vi "JOYSTICK MANUAL SUBVI.vi"   [LabVIEW 2013]
uses:
  <vilib>/Rock Robotics/WPI/Joystick/WPI_JoystickGetSetRefNum.vi
types:
  T1 = typedef "WPI_JoystickDevRef.ctl" = cluster{"Device":T2}
  T2 = typedef "WPI_JoystickDeviceEnum.ctl" = enum16{"USB 1", "USB 2", "USB 3", "USB 4", "Kinect 1", "Kinect 2"}
  T3 = cluster{"axis 1 (x)":dbl, "axis 2 (y)":dbl, "axis 3 (throttle)":dbl, "axis 4":dbl, "axis 5":dbl, "axis 6":dbl}
  T4 = typedef "WPI_JoystickButtonState.ctl" = cluster{"Button 1":bool, "Button 2":bool, "Button 3":bool, "Button 4":bool, "Button 5":bool, "Button 6":bool, "Button 7":bool, "Button 8":bool, "Button 9":bool, "Button 10":bool, "Button 11":bool, "Button 12":bool}
  T5 = typedef "WPI_MotorControlDeviceRef.ctl" = cluster{"DeviceStatus":errorcluster, "Type":enum16{"PWM", "CAN"}, "PWM":cluster{"Digital Module":T6, "PWM Channel":T7, "DeadBand":T8}, "CAN":cluster{"Device Number":u8, "Control Mode":T9, "Semaphore":T10, "Max Vout":dbl}, "Invert":bool, "TransformRef":T11, "InvTransformRef":T11}
  T6 = typedef "FPGA_TypedefDigitalModule.ctl" = enum16{"Digital Module 1", "Digital Module 2"}
  T7 = typedef "FPGA_DIOPWMChannel.ctl" = enum8{"PWM 1", "PWM 2", "PWM 3", "PWM 4", "PWM 5", "PWM 6", "PWM 7", "PWM 8", "PWM 9", "PWM 10", "Invalid"}
  T8 = typedef "WPI_PWMDeadband.ctl" = cluster{"Name":string, "maxPositivePwm":i32, "minPositivePwm":i32, "centerPwm":i32, "maxNegativePwm":i32, "minNegativePwm":i32, "angularRange":u16}
  T9 = typedef "WPI_CANJaguar_ControlMode.ctl" = enum8{"Percent VBus", "Current", "Speed", "Position", "Voltage"}
  T10 = typedef "Semaphore RefNum" = refnum<k1>
  T11 = typedef "WPI_PWMTransform_ConPane.ctl" = refnum<vi>
  T12 = typedef "WPI_DigitalInputDevRef.ctl" = cluster{"DevStatus":errorcluster, "DIO Channel":T13, "Digital Module":T6}
  T13 = typedef "FPGA_DIOChannel.ctl" = enum8{"DIO 1", "DIO 2", "DIO 3", "DIO 4", "DIO 5", "DIO 6", "DIO 7", "DIO 8", "DIO 9", "DIO 10", "DIO 11", "DIO 12", "DIO 13", "DIO 14", "Invalid"}
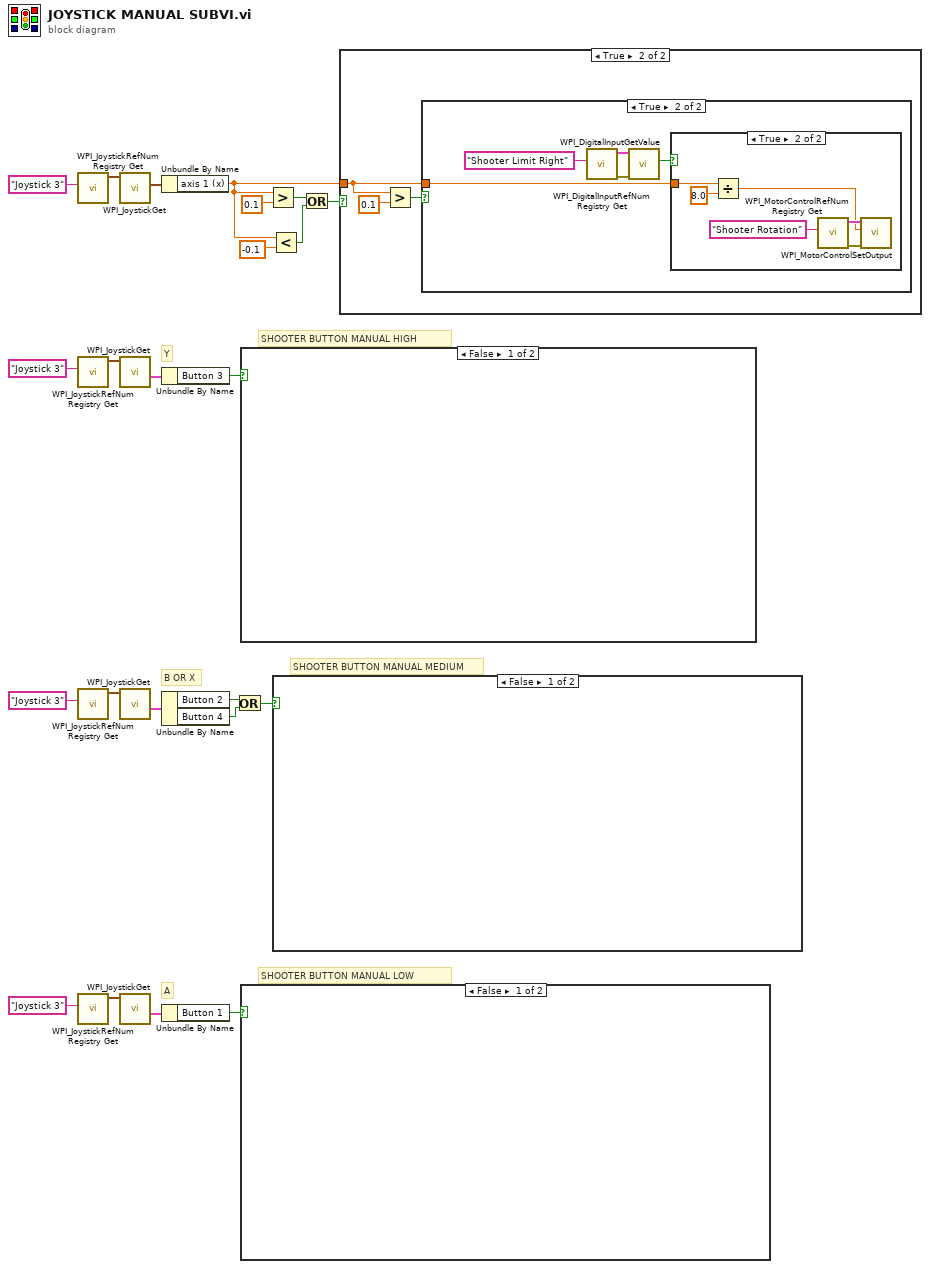
[diagram p0: block diagram]
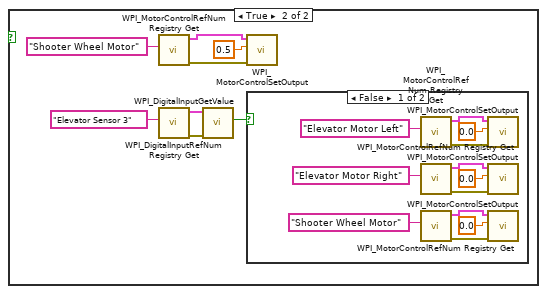
[diagram p2: hidden frame]
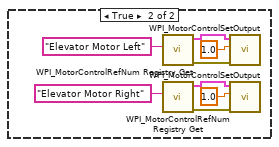
[diagram p3: hidden frame]
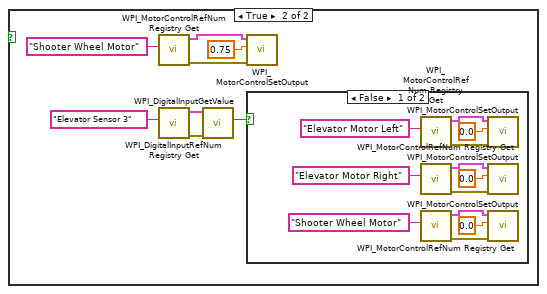
[diagram p4: hidden frame]
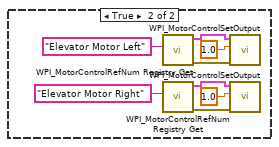
[diagram p5: hidden frame]
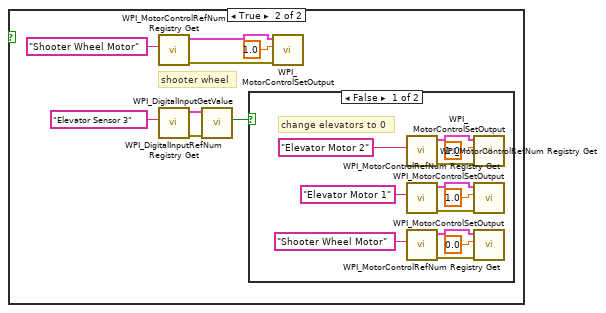
[diagram p6: hidden frame]
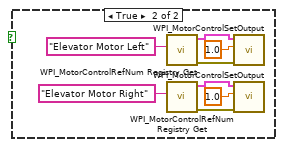
[diagram p7: hidden frame]
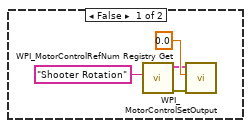
[diagram p8: hidden frame]
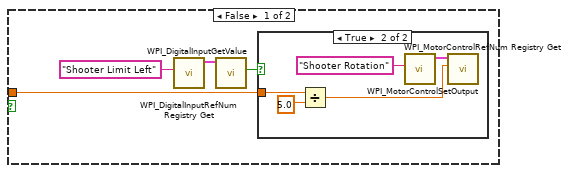
[diagram p9: hidden frame]
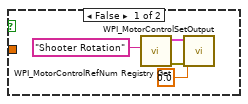
[diagram p10: hidden frame]
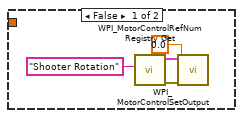
[diagram p11: hidden frame]
diagram:
  # "A"
  # "SHOOTER BUTTON MANUAL LOW"
  # "B OR X"
  # "SHOOTER BUTTON MANUAL MEDIUM"
  # "Y"
  # "SHOOTER BUTTON MANUAL HIGH"
  n1 = call <vilib>:"WPI_JoystickRefNum Registry Get.vi"("refnum name"="Joystick 3") -> ("JoystickDevRef"=w15:T1)  [unwired: 9 in, 1 out]
  n2 = call <vilib>:"WPI_JoystickRefNum Registry Get.vi"("refnum name"="Joystick 3") -> ("JoystickDevRef"=w14:T1)  [unwired: 9 in, 1 out]
  n3 = call <vilib>:"WPI_JoystickRefNum Registry Get.vi"("refnum name"="Joystick 3") -> ("JoystickDevRef"=w10:T1)  [unwired: 9 in, 1 out]
  n4 = call <vilib>:"WPI_JoystickRefNum Registry Get.vi"("refnum name"="Joystick 3") -> ("JoystickDevRef"=w4:T1)  [unwired: 9 in, 1 out]
  n5 = call <vilib>:"WPI_JoystickGet.vi"("JoystickDevRef"=w15) -> ("Axes"=w17:T3)  [unwired: 4 in, 2 out]
  n6 = call <vilib>:"WPI_JoystickGet.vi"("JoystickDevRef"=w14) -> ("Buttons"=w13:T4)  [unwired: 4 in, 2 out]
  n7 = call <vilib>:"WPI_JoystickGet.vi"("JoystickDevRef"=w10) -> ("Buttons"=w8:T4)  [unwired: 4 in, 2 out]
  n8 = call <vilib>:"WPI_JoystickGet.vi"("JoystickDevRef"=w4) -> ("Buttons"=w2:T4)  [unwired: 4 in, 2 out]
  n9 = Unbundle By Name(w17) -> ("axis 1 (x)"=w21:dbl)
  n10 = Unbundle By Name(w13) -> ("Button 3"=w12:bool)
  n11 = Unbundle By Name(w8) -> ("Button 2"=w7:bool, "Button 4"=w6:bool)
  n12 = Unbundle By Name(w2) -> ("Button 1"=w1:bool)
  n13 = Or(x=w7, y=w6) -> (x .or. y?=w5:bool)
  n14 = case shown="False" w12 {
    frame False {
    }
    frame True {
      # "shooter wheel"
      n15 = call <vilib>:"WPI_MotorControlRefNum Registry Get.vi"("refnum name"="Shooter Wheel Motor") -> ("error out"=w27:errorcluster, "MotorControlDevRef"=w26:T5)  [unwired: 9 in]
      n16 = call <vilib>:"WPI_DigitalInputRefNum Registry Get.vi"("refnum name"="Elevator Sensor 3") -> ("error out"=w30:errorcluster, "DigitalInputDevRef"=w29:T12)  [unwired: 9 in]
      n17 = call <vilib>:"WPI_DigitalInputGetValue.vi"("error in (no error)"=w30, "DigitalInputDevRef"=w29) -> ("Value"=w28:bool)  [unwired: 7 in, 2 out]
      n18 = case shown="False" w28 {
        frame False {
          # "change elevators to 0"
          n19 = call <vilib>:"WPI_MotorControlRefNum Registry Get.vi"("refnum name"="Elevator Motor 2") -> ("error out"=w43:errorcluster, "MotorControlDevRef"=w42:T5)  [unwired: 9 in]
          n20 = call <vilib>:"WPI_MotorControlRefNum Registry Get.vi"("refnum name"="Elevator Motor 1") -> ("error out"=w39:errorcluster, "MotorControlDevRef"=w38:T5)  [unwired: 9 in]
          n21 = call <vilib>:"WPI_MotorControlRefNum Registry Get.vi"("refnum name"="Shooter Wheel Motor") -> ("error out"=w35:errorcluster, "MotorControlDevRef"=w34:T5)  [unwired: 9 in]
          n22 = call <vilib>:"WPI_MotorControlSetOutput.vi"("error in (no error)"=w43, "Output"=1.0, "MotorControlDevRef"=w42) -> ()  [unwired: 6 in, 3 out]
          n23 = call <vilib>:"WPI_MotorControlSetOutput.vi"("error in (no error)"=w39, "Output"=1.0, "MotorControlDevRef"=w38) -> ()  [unwired: 6 in, 3 out]
          n24 = call <vilib>:"WPI_MotorControlSetOutput.vi"("error in (no error)"=w35, "Output"=0.0, "MotorControlDevRef"=w34) -> ()  [unwired: 6 in, 3 out]
        }
        frame True {
          n25 = call <vilib>:"WPI_MotorControlRefNum Registry Get.vi"("refnum name"="Elevator Motor Left") -> ("error out"=w51:errorcluster, "MotorControlDevRef"=w50:T5)  [unwired: 9 in]
          n26 = call <vilib>:"WPI_MotorControlRefNum Registry Get.vi"("refnum name"="Elevator Motor Right") -> ("error out"=w47:errorcluster, "MotorControlDevRef"=w46:T5)  [unwired: 9 in]
          n27 = call <vilib>:"WPI_MotorControlSetOutput.vi"("error in (no error)"=w51, "Output"=1.0, "MotorControlDevRef"=w50) -> ()  [unwired: 6 in, 3 out]
          n28 = call <vilib>:"WPI_MotorControlSetOutput.vi"("error in (no error)"=w47, "Output"=1.0, "MotorControlDevRef"=w46) -> ()  [unwired: 6 in, 3 out]
        }
      }
      n29 = call <vilib>:"WPI_MotorControlSetOutput.vi"("error in (no error)"=w27, "Output"=1.0, "MotorControlDevRef"=w26) -> ()  [unwired: 6 in, 3 out]
    }
  }
  n30 = case shown="False" w1 {
    frame False {
    }
    frame True {
      n31 = call <vilib>:"WPI_MotorControlRefNum Registry Get.vi"("refnum name"="Shooter Wheel Motor") -> ("error out"=w55:errorcluster, "MotorControlDevRef"=w54:T5)  [unwired: 9 in]
      n32 = call <vilib>:"WPI_DigitalInputRefNum Registry Get.vi"("refnum name"="Elevator Sensor 3") -> ("error out"=w58:errorcluster, "DigitalInputDevRef"=w57:T12)  [unwired: 9 in]
      n33 = call <vilib>:"WPI_DigitalInputGetValue.vi"("error in (no error)"=w58, "DigitalInputDevRef"=w57) -> ("Value"=w56:bool)  [unwired: 7 in, 2 out]
      n34 = call <vilib>:"WPI_MotorControlSetOutput.vi"("error in (no error)"=w55, "Output"=0.5, "MotorControlDevRef"=w54) -> ()  [unwired: 6 in, 3 out]
      n35 = case shown="False" w56 {
        frame False {
          n36 = call <vilib>:"WPI_MotorControlRefNum Registry Get.vi"("refnum name"="Elevator Motor Left") -> ("error out"=w71:errorcluster, "MotorControlDevRef"=w70:T5)  [unwired: 9 in]
          n37 = call <vilib>:"WPI_MotorControlRefNum Registry Get.vi"("refnum name"="Elevator Motor Right") -> ("error out"=w67:errorcluster, "MotorControlDevRef"=w66:T5)  [unwired: 9 in]
          n38 = call <vilib>:"WPI_MotorControlRefNum Registry Get.vi"("refnum name"="Shooter Wheel Motor") -> ("error out"=w63:errorcluster, "MotorControlDevRef"=w62:T5)  [unwired: 9 in]
          n39 = call <vilib>:"WPI_MotorControlSetOutput.vi"("error in (no error)"=w71, "Output"=0.0, "MotorControlDevRef"=w70) -> ()  [unwired: 6 in, 3 out]
          n40 = call <vilib>:"WPI_MotorControlSetOutput.vi"("error in (no error)"=w67, "Output"=0.0, "MotorControlDevRef"=w66) -> ()  [unwired: 6 in, 3 out]
          n41 = call <vilib>:"WPI_MotorControlSetOutput.vi"("error in (no error)"=w63, "Output"=0.0, "MotorControlDevRef"=w62) -> ()  [unwired: 6 in, 3 out]
        }
        frame True {
          n42 = call <vilib>:"WPI_MotorControlRefNum Registry Get.vi"("refnum name"="Elevator Motor Left") -> ("error out"=w79:errorcluster, "MotorControlDevRef"=w78:T5)  [unwired: 9 in]
          n43 = call <vilib>:"WPI_MotorControlRefNum Registry Get.vi"("refnum name"="Elevator Motor Right") -> ("error out"=w75:errorcluster, "MotorControlDevRef"=w74:T5)  [unwired: 9 in]
          n44 = call <vilib>:"WPI_MotorControlSetOutput.vi"("error in (no error)"=w79, "Output"=1.0, "MotorControlDevRef"=w78) -> ()  [unwired: 6 in, 3 out]
          n45 = call <vilib>:"WPI_MotorControlSetOutput.vi"("error in (no error)"=w75, "Output"=1.0, "MotorControlDevRef"=w74) -> ()  [unwired: 6 in, 3 out]
        }
      }
    }
  }
  n46 = Greater?(x=w21, y=0.1) -> (0:w22:bool)
  n47 = Less?(x=w21, y=-0.1) -> (x < y?=w23:bool)
  n48 = case shown="False" w5 {
    frame False {
    }
    frame True {
      n49 = call <vilib>:"WPI_MotorControlRefNum Registry Get.vi"("refnum name"="Shooter Wheel Motor") -> ("error out"=w83:errorcluster, "MotorControlDevRef"=w82:T5)  [unwired: 9 in]
      n50 = call <vilib>:"WPI_DigitalInputRefNum Registry Get.vi"("refnum name"="Elevator Sensor 3") -> ("error out"=w86:errorcluster, "DigitalInputDevRef"=w85:T12)  [unwired: 9 in]
      n51 = call <vilib>:"WPI_DigitalInputGetValue.vi"("error in (no error)"=w86, "DigitalInputDevRef"=w85) -> ("Value"=w84:bool)  [unwired: 7 in, 2 out]
      n52 = call <vilib>:"WPI_MotorControlSetOutput.vi"("error in (no error)"=w83, "Output"=0.75, "MotorControlDevRef"=w82) -> ()  [unwired: 6 in, 3 out]
      n53 = case shown="False" w84 {
        frame False {
          n54 = call <vilib>:"WPI_MotorControlRefNum Registry Get.vi"("refnum name"="Elevator Motor Left") -> ("error out"=w99:errorcluster, "MotorControlDevRef"=w98:T5)  [unwired: 9 in]
          n55 = call <vilib>:"WPI_MotorControlRefNum Registry Get.vi"("refnum name"="Elevator Motor Right") -> ("error out"=w95:errorcluster, "MotorControlDevRef"=w94:T5)  [unwired: 9 in]
          n56 = call <vilib>:"WPI_MotorControlRefNum Registry Get.vi"("refnum name"="Shooter Wheel Motor") -> ("error out"=w91:errorcluster, "MotorControlDevRef"=w90:T5)  [unwired: 9 in]
          n57 = call <vilib>:"WPI_MotorControlSetOutput.vi"("error in (no error)"=w99, "Output"=0.0, "MotorControlDevRef"=w98) -> ()  [unwired: 6 in, 3 out]
          n58 = call <vilib>:"WPI_MotorControlSetOutput.vi"("error in (no error)"=w95, "Output"=0.0, "MotorControlDevRef"=w94) -> ()  [unwired: 6 in, 3 out]
          n59 = call <vilib>:"WPI_MotorControlSetOutput.vi"("error in (no error)"=w91, "Output"=0.0, "MotorControlDevRef"=w90) -> ()  [unwired: 6 in, 3 out]
        }
        frame True {
          n60 = call <vilib>:"WPI_MotorControlRefNum Registry Get.vi"("refnum name"="Elevator Motor Left") -> ("error out"=w107:errorcluster, "MotorControlDevRef"=w106:T5)  [unwired: 9 in]
          n61 = call <vilib>:"WPI_MotorControlRefNum Registry Get.vi"("refnum name"="Elevator Motor Right") -> ("error out"=w103:errorcluster, "MotorControlDevRef"=w102:T5)  [unwired: 9 in]
          n62 = call <vilib>:"WPI_MotorControlSetOutput.vi"("error in (no error)"=w107, "Output"=1.0, "MotorControlDevRef"=w106) -> ()  [unwired: 6 in, 3 out]
          n63 = call <vilib>:"WPI_MotorControlSetOutput.vi"("error in (no error)"=w103, "Output"=1.0, "MotorControlDevRef"=w102) -> ()  [unwired: 6 in, 3 out]
        }
      }
    }
  }
  n64 = Or(x=w22, y=w23) -> (x .or. y?=w19:bool)
  n65 = case shown="True" w19 {
    tunnel: w21 -> [_ w112]
    frame False {
      n66 = call <vilib>:"WPI_MotorControlRefNum Registry Get.vi"("refnum name"="Shooter Rotation") -> ("error out"=w111:errorcluster, "MotorControlDevRef"=w109:T5)  [unwired: 9 in]
      n67 = call <vilib>:"WPI_MotorControlSetOutput.vi"("error in (no error)"=w111, "Output"=0.0, "MotorControlDevRef"=w109) -> ()  [unwired: 6 in, 3 out]
    }
    frame True {
      n68 = Greater?(x=w112, y=0.1) -> (0:w113:bool)
      n69 = case shown="True" w113 {
        tunnel: w112 -> [w116 w132]
        frame False {
          n70 = call <vilib>:"WPI_DigitalInputRefNum Registry Get.vi"("refnum name"="Shooter Limit Left") -> ("DigitalInputDevRef"=w117:T12)  [unwired: 9 in, 1 out]
          n71 = call <vilib>:"WPI_DigitalInputGetValue.vi"("DigitalInputDevRef"=w117) -> ("Value"=w115:bool)  [unwired: 8 in, 2 out]
          n72 = case shown="True" w115 {
            tunnel: w116 -> [_ w123]
            frame False {
              n73 = call <vilib>:"WPI_MotorControlRefNum Registry Get.vi"("refnum name"="Shooter Rotation") -> ("error out"=w119:errorcluster, "MotorControlDevRef"=w122:T5)  [unwired: 9 in]
              n74 = call <vilib>:"WPI_MotorControlSetOutput.vi"("error in (no error)"=w119, "Output"=0.0, "MotorControlDevRef"=w122) -> ()  [unwired: 6 in, 3 out]
            }
            frame True {
              n75 = Divide(x=w123, y=5.0) -> (x/y=w125:dbl)
              n76 = call <vilib>:"WPI_MotorControlRefNum Registry Get.vi"("refnum name"="Shooter Rotation") -> ("MotorControlDevRef"=w127:T5)  [unwired: 9 in, 1 out]
              n77 = call <vilib>:"WPI_MotorControlSetOutput.vi"("Output"=w125, "MotorControlDevRef"=w127) -> ()  [unwired: 7 in, 3 out]
            }
          }
        }
        frame True {
          n78 = call <vilib>:"WPI_DigitalInputRefNum Registry Get.vi"("refnum name"="Shooter Limit Right") -> ("error out"=w128:errorcluster, "DigitalInputDevRef"=w129:T12)  [unwired: 9 in]
          n79 = call <vilib>:"WPI_DigitalInputGetValue.vi"("error in (no error)"=w128, "DigitalInputDevRef"=w129) -> ("Value"=w130:bool)  [unwired: 7 in, 2 out]
          n80 = case shown="True" w130 {
            tunnel: w132 -> [_ w137]
            frame False {
              n81 = call <vilib>:"WPI_MotorControlRefNum Registry Get.vi"("refnum name"="Shooter Rotation") -> ("error out"=w135:errorcluster, "MotorControlDevRef"=w136:T5)  [unwired: 9 in]
              n82 = call <vilib>:"WPI_MotorControlSetOutput.vi"("error in (no error)"=w135, "Output"=0.0, "MotorControlDevRef"=w136) -> ()  [unwired: 6 in, 3 out]
            }
            frame True {
              n83 = Divide(x=w137, y=8.0) -> (x/y=w138:dbl)
              n84 = call <vilib>:"WPI_MotorControlRefNum Registry Get.vi"("refnum name"="Shooter Rotation") -> ("error out"=w141:errorcluster, "MotorControlDevRef"=w142:T5)  [unwired: 9 in]
              n85 = call <vilib>:"WPI_MotorControlSetOutput.vi"("error in (no error)"=w141, "Output"=w138, "MotorControlDevRef"=w142) -> ()  [unwired: 6 in, 3 out]
            }
          }
        }
      }
    }
  }
